vi "Start Panel.vi"(7 "Project In":refnum<class "Project.lvclass">, 8 "error in (no error)":errorcluster, 9 "Panel Host":refnum<vi>, 10 "Panel":enum16{"UI Setting Panel", "Output Panel"}(ring), 11 "UIStep in":refnum<class "UIStep.lvclass">) -> (0 "error out":errorcluster, 1 "Panel VI out":refnum<vi>, 3 "UIStep out":refnum<class "UIStep.lvclass">)   [LabVIEW 2015, in "UIStep.lvclass"]
uses:
  UIStep.lvclass
  Project.lvclass
  Step.lvclass
  OutputUI/Output Panel.vi
  UIStep Setting Panel.vi
  OutputUI.lvclass
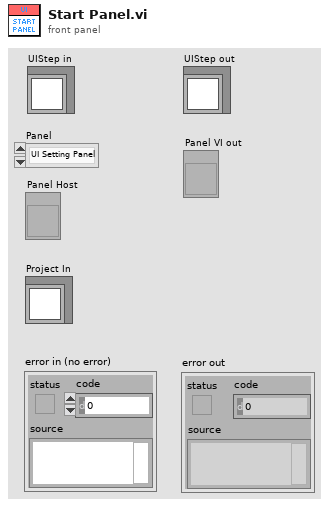
[diagram p1: front panel]
types:
  T1 = enum32{"Invalid", "Standard", "Closed", "Hidden", "Minimized", "Maximized"}
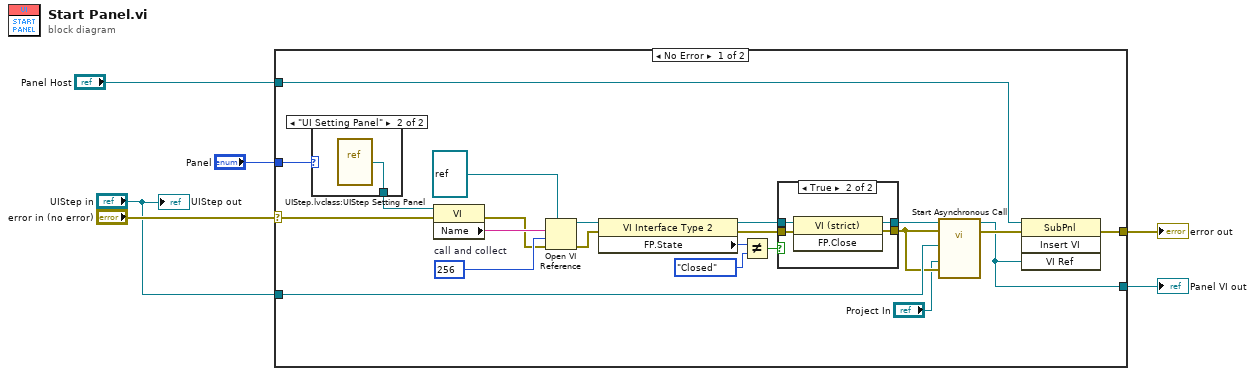
[diagram p0: block diagram]
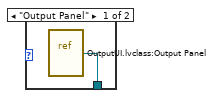
[diagram p2: hidden frame]
diagram:
  n1 = case shown="No Error" "error in (no error)" {
    selector: "error in (no error)" -> [w28 w37]
    tunnel: [w27 w37] -> w5
    tunnel: "UIStep in" -> [w26 _]
    tunnel: "Panel Host" -> [w10 _]
    tunnel: [w9 _] -> w3
    tunnel: "Panel" -> [w8 _]
    frame No Error {
      w22 = 256  # call and collect
      n2 = case shown="\"UI Setting Panel\"" w8 {
        tunnel: [w29 w30] -> w25
        frame "Output Panel" {
          n3 = vi-ref "OutputUI.lvclass:Output Panel.vi"() -> (w29:refnum<vi>)
        }
        frame "UI Setting Panel" {
          n4 = vi-ref "UIStep.lvclass:UIStep Setting Panel.vi"() -> (w30:refnum<vi>)
        }
      }
      n5 = property class="VI"(reference=w25, error in=w28) -> (error out=w20:errorcluster, "Name"=w23:string)  [unwired: 1 out]
      n6 = Open VI Reference(type specifier VI Refnum (for type only)=refnum<vi> refnum, vi path=w23, options=w22, error in (no error)=w20) -> (vi reference=w14:refnum<vi>, error out=w13:errorcluster)  [unwired: 2 in]
      n7 = property class="VI Interface Type 2"(reference=w14, error in=w13) -> (reference out=w18:refnum<vi>, error out=w19:errorcluster, "FP.State"=w15:T1)
      n8 = Not Equal?(x=w15, y=T1."Closed" ("Front Panel Window:State")) -> (x != y?=w17:bool)
      n9 = case shown="True" w17 {
        tunnel: w18 -> [w32 w36]
        tunnel: w19 -> [w31 w35]
        tunnel: [w32 w34] -> w12
        tunnel: [w31 w33] -> w11
        frame False {
        }
        frame True {
          n10 = invoke class="VI (strict)" method="FP.Close"(reference=w36, error in=w35) -> (reference out=w34:refnum<vi>, error out=w33:errorcluster)  [unwired: 1 in, 1 out]
        }
      }
      n11 = call-by-ref "Start Asynchronous Call"(reference=w12, error in=w11, 8:"error in (no error)"=w11, "Project In"="Project In", "Step in"=w26) -> (reference out=w9:refnum<vi>, error out=w21:errorcluster)  [unwired: 7 in, 2 out]
      n12 = invoke class="SubPnl" method="Insert VI"(reference=w10, error in=w21, "VI Ref"=w9) -> (error out=w27:errorcluster)  [unwired: 1 in, 3 out]
    }
    frame Error {
    }
  }
  "error out" <- w5
  "Panel VI out" <- w3
  "UIStep out" <- "UIStep in"
